vi "PH_Beckhoff_Common.create BB Tagnameset.vi"(1 "#":i32, 2 "Instance Name":string) -> (0 "output cluster":T1={"Sensor Remote controlled"="N/A", "Sensor Out"="N/A", "Sensor In"="N/A", "Actor Direction In"="N/A", "Actor Move"="N/A", "Sensor Power ok"="N/A", "Instance"="N/A"})   [LabVIEW 2014, in "PH_Beckhoff_Common.lvlib"]
uses:
  PH_Beckhoff_Common.lvlib
  PH_Beckhoff_Common.BB Tagnames.ctl
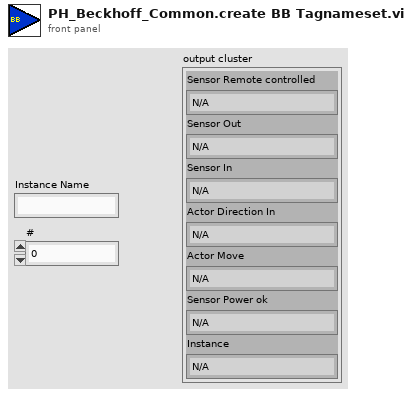
[diagram p1: front panel]
types:
  T1 = typedef "PH_Beckhoff_Common.lvlib/PH_Beckhoff_Common.BB Tagnames.ctl" = cluster{"Sensor Remote controlled":string, "Sensor Out":string, "Sensor In":string, "Actor Direction In":string, "Actor Move":string, "Sensor Power ok":string, "Instance":string}
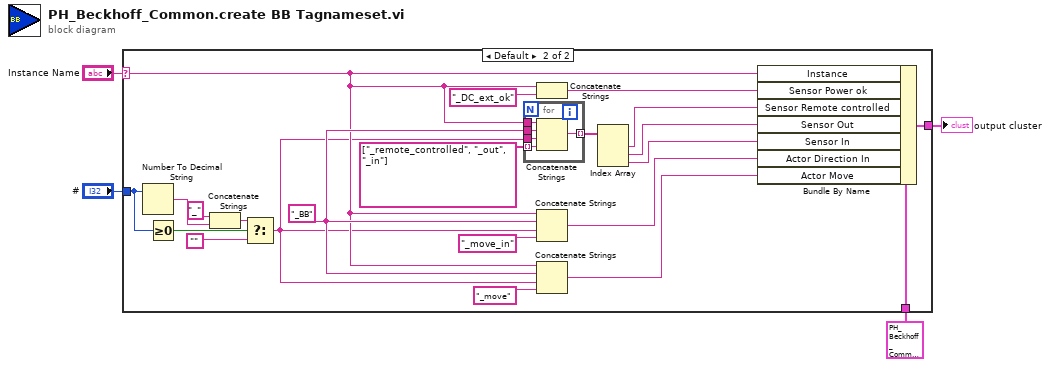
[diagram p0: block diagram]
diagram:
  n1 = case shown="Default" "Instance Name" {
    selector: "Instance Name" -> [_ w13]
    tunnel: "#" -> [_ w12]
    tunnel: T1 {"Sensor Remote controlled"="N/A", "Sensor Out"="N/A", "Sensor In"="N/A", "Actor Direction In"="N/A", "Actor Move"="N/A", "Sensor Power ok"="N/A", "Instance"="N/A"} ("BB Tags") -> [w5 w21]
    tunnel: [w5 w20] -> w2
    frame "", "N/A" {
    }
    frame Default {
      w19 = "_BB" ("string")
      n2 = Number To Decimal String(number=w12) -> (decimal integer string=w7:string)  [unwired: 1 in]
      n3 = Greater Or Equal To 0?(x=w12) -> (x >= 0?=w10:bool)
      n4 = Concatenate Strings("_" ("string"), w7) -> (w9:string)
      n5 = Select(t=w9, s=w10, f="") -> (s? t:f=w6:string)
      n6 = for {
        tunnel: w13 -> [w32]
        tunnel: [w31] -> w18 mode=indexing
        tunnel: string[] ["_remote_controlled", "_out", "_in"] -> [w30] mode=indexing
        tunnel: w6 -> [w29]
        tunnel: w19 -> [w28]
        n7 = Concatenate Strings(w32, w28, w29, w30) -> (w31:string)
      }
      n8 = Concatenate Strings(w13, "_DC_ext_ok" ("string")) -> (w22:string)
      n9 = Concatenate Strings(w13, w19, w6, "_move_in") -> (w24:string)
      n10 = Concatenate Strings(w13, w19, w6, "_move") -> (w23:string)
      n11 = Index Array(array=w18) -> (element #1=w27:string, element #2=w26:string, element #3=w25:string)  [unwired: 3 in]
      n12 = Bundle By Name(cluster=w21, "Instance"=w13, "Sensor Power ok"=w22, "Sensor Remote controlled"=w27, "Sensor Out"=w26, "Sensor In"=w25, "Actor Direction In"=w24, "Actor Move"=w23) -> (w20:T1)
    }
  }
  "output cluster" <- w2
